vi "Decrypt_Selected_File_of_CryptedFolder.vi"(8 "error in (no error)":errorcluster, 10 "relative path":string, 11 "object in":refnum<class "Crypter.lvclass">) -> (0 "error out":errorcluster, 2 "Dencrypted text":string, 3 "object out":refnum<class "Crypter.lvclass">)   [LabVIEW 2016, in "Crypter.lvclass"]
uses:
  Crypter.lvclass
  Crypter.lvclass/Crypter.ctl
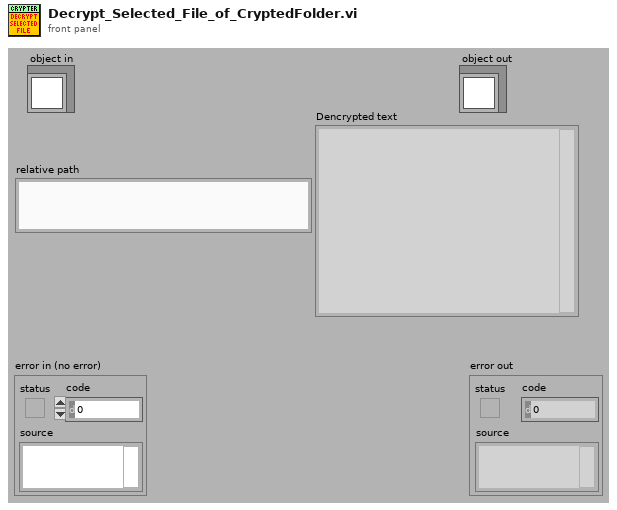
[diagram p1: front panel]
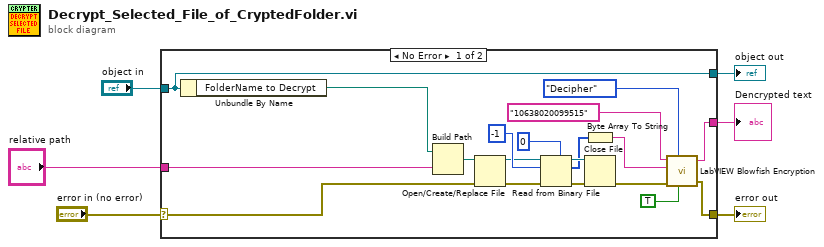
[diagram p0: block diagram]
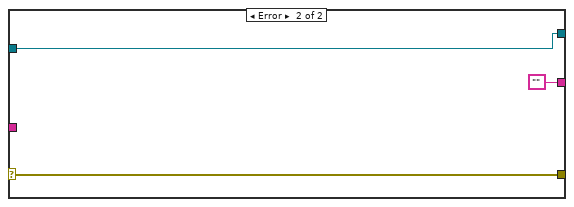
[diagram p2: hidden frame]
diagram:
  n1 = case shown="No Error" "error in (no error)" {
    selector: "error in (no error)" -> [w12 w28]
    tunnel: [w11 w28] -> w5
    tunnel: [w25 w27] -> w3
    tunnel: "object in" -> [w25 w27]
    tunnel: [w13 ""] -> w2
    tunnel: "relative path" -> [w8 _]
    frame No Error {
      n2 = Unbundle By Name(w25) -> ("FolderName to Decrypt"=w24:path)
      n3 = Build Path(base path=w24, name or relative path=w8) -> (appended path=w14:path)
      n4 = Open/Create/Replace File(file path (use dialog)=w14, error in=w12) -> (refnum out=w16:refnum<file>, error out=w18:errorcluster)  [unwired: 4 in, 1 out]
      n5 = Read from Binary File(5:u8 0, 8:w18, 10:-1 ("count (1)"), 11:w16) -> (0:w17:errorcluster, 2:w10:u8[], 3:w15:refnum<file>)  [unwired: 2 in, 1 out]
      n6 = Byte Array To String(unsigned byte array=w10) -> (string=w9:string)
      n7 = Close File(refnum=w15, error in=w17) -> (error out=w21:errorcluster)  [unwired: 1 out]
      n8 = call "LabVIEW Blowfish Encryption.vi"("Password"="10638020099515", "Enc/Dec"=enum16{"Encipher", "Decipher"}."Decipher", "Input Text"=w9, "Output As ASCII\nfor email Transmission"=TRUE ("Output As ASCII\nfor email Transmission"), "error in (no error)"=w21) -> ("Output text"=w13:string, "error out"=w11:errorcluster)  [unwired: 1 in, 1 out]
    }
    frame Error {
    }
  }
  "error out" <- w5
  "object out" <- w3
  "Dencrypted text" <- w2
